vi "Transformationto360x360matrixcoordinates_171213.vi"(11 "FilteredInputData":dbl[][](array[numeric])) -> (2 "360Y":dbl[](array[numeric]), 3 "360X":dbl[](array[numeric]))   [LabVIEW 2016]
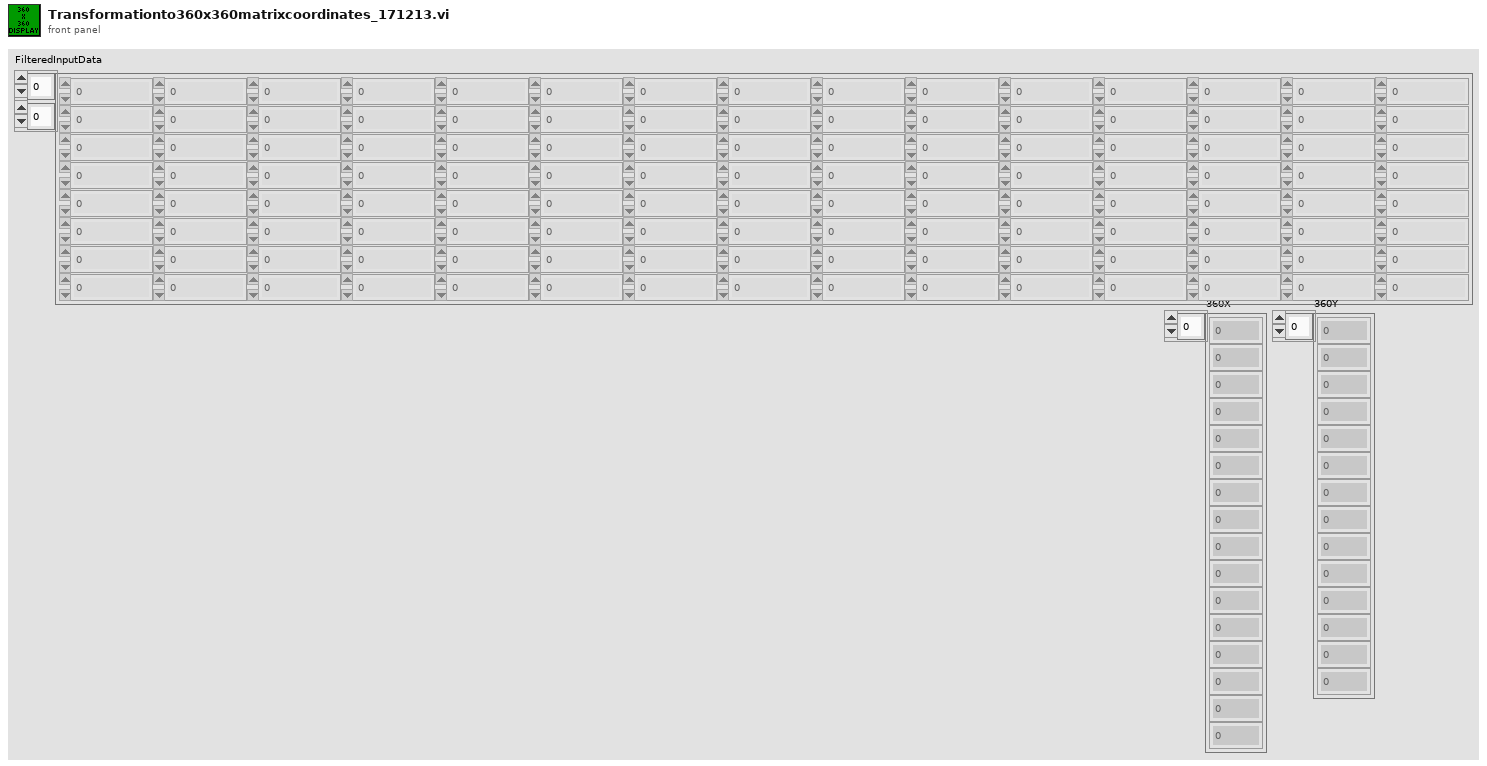
[diagram p1: front panel]
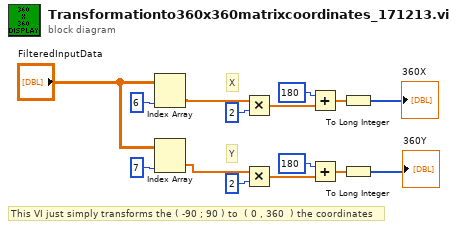
[diagram p0: block diagram]
diagram:
  # "Y"
  # "X"
  # "This VI just simply transforms the ( -90 ; 90 ) to  ( 0 , 360  ) the coordinates"
  n1 = Index Array(array="FilteredInputData", index (col)=6 ("disabled index (col)")) -> (element=w4:dbl[])  [unwired: 1 in]
  n2 = Index Array(array="FilteredInputData", index (col)=7 ("disabled index (col)")) -> (element=w3:dbl[])  [unwired: 1 in]
  n3 = Multiply(x=w4, y=2 ("disabled index (col)")) -> (x*y=w7:dbl[])
  n4 = Multiply(x=w3, y=2 ("disabled index (col)")) -> (x*y=w8:dbl[])
  n5 = Add(x=180 ("disabled index (col)"), y=w7) -> (x+y=w12:dbl[])
  n6 = Add(x=180 ("disabled index (col)"), y=w8) -> (x+y=w11:dbl[])
  n7 = To Long Integer(number=w12) -> (32bit integer=→"360X":i32[])
  n8 = To Long Integer(number=w11) -> (32bit integer=→"360Y":i32[])
